vi "Magazine Control 3.0.vi"(0 "Magazine Overflow Power":dbl=1.0, 4 "Magazine Power":dbl=1.0, 6 "Intake Power":dbl=1.0, 8 "Outtake Sensor":bool, 9 "Intake Sensor":bool, 10 "Outtake Button":bool, 11 "Intake Button":bool) -> (2 "Magazine":dbl, 3 "Intake":dbl)   [LabVIEW 2019]
uses:
  Magazine State.ctl
  78d4d847-6c27-4930-b494-8e57f4631178.vi
  83c46ad4-0f57-42ca-80be-7e1131384452.vi
  952471bd-31fd-4431-ad26-f7d2215ef338.vi
panel:
  out "Current State":T1
  in  "Initial State":T1
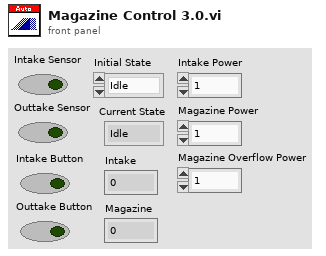
[diagram p1: front panel]
types:
  T1 = typedef "Magazine State.ctl" = enum16{"Idle", "Intake Idle", "Move Cell", "Prevent Overflow", "Outtake Idle", "Shoot"}
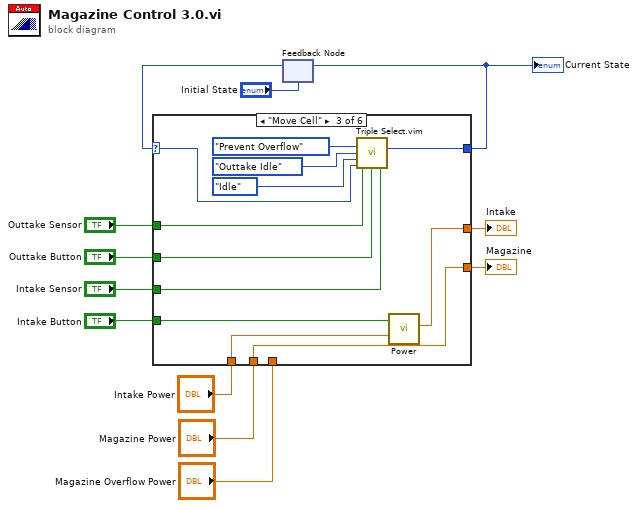
[diagram p0: block diagram]
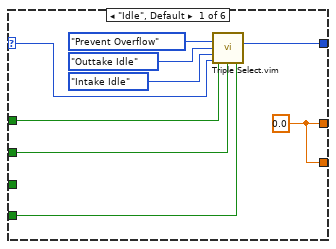
[diagram p2: hidden frame]
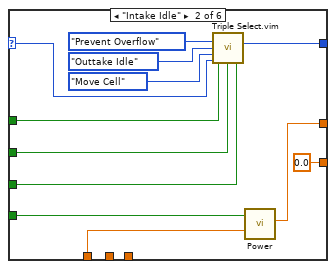
[diagram p3: hidden frame]
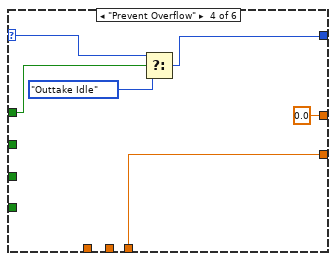
[diagram p4: hidden frame]
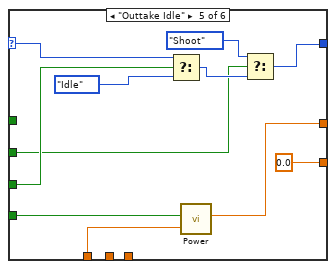
[diagram p5: hidden frame]
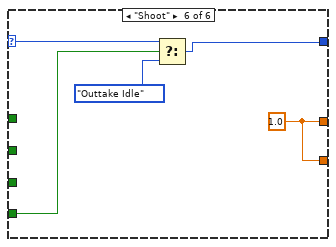
[diagram p6: hidden frame]
diagram:
  n1 = feedback #1("Initial State") -> (w3:T1)
  n2 = case shown="\"Move Cell\"" w3 {
    selector: w3 -> [w13 w27 w39 w49 w58 w66]
    tunnel: "Intake Button" -> [w17 w31 w45 _ w62 w67]
    tunnel: [w21 w33 w44 0.0 ("Output") w61 w63] -> w10
    tunnel: [w21 0.0 w43 w51 0.0 ("Magazine Overflow Power") w63] -> w9
    tunnel: "Intake Power" -> [_ w22 w34 _ w52 _]
    tunnel: "Intake Sensor" -> [_ w24 w36 _ w59 _]
    tunnel: "Magazine Power" -> [_ _ w43 _ _ _]
    tunnel: [w14 w23 w35 w48 w53 w64] -> w1
    tunnel: "Magazine Overflow Power" -> [_ _ _ w51 _ _]
    tunnel: "Outtake Button" -> [w16 w26 w37 _ w55 _]
    tunnel: "Outtake Sensor" -> [w15 w25 w38 w46 _ _]
    frame "Idle", Default {
      w21 = 0.0
      n3 = call "Triple Select.vim"("Input 1"=Magazine_State."Prevent Overflow" ("lower limit"), "Input 2"=Magazine_State."Outtake Idle" ("lower limit"), "Input 3"=Magazine_State."Intake Idle", "Input 4"=w13, "Selection 1"=w15, "Selection 2"=w16, "Selection 3"=w17) -> ("Output"=w14:T1)  [unwired: 8 in]
    }
    frame "Intake Idle" {
      n4 = call "Triple Select.vim"("Input 1"=Magazine_State."Prevent Overflow" ("lower limit"), "Input 2"=Magazine_State."Outtake Idle" ("lower limit"), "Input 3"=Magazine_State."Move Cell", "Input 4"=w27, "Selection 1"=w25, "Selection 2"=w26, "Selection 3"=w24) -> ("Output"=w23:T1)  [unwired: 8 in]
      n5 = call "Power.vi"("Positive Power"=w22, "Positive"=w31) -> ("Output"=w33:dbl)  [unwired: 9 in]
    }
    frame "Move Cell" {
      n6 = call "Triple Select.vim"("Input 1"=Magazine_State."Prevent Overflow" ("lower limit"), "Input 2"=Magazine_State."Outtake Idle" ("lower limit"), "Input 3"=Magazine_State."Idle", "Input 4"=w39, "Selection 1"=w38, "Selection 2"=w37, "Selection 3"=w36) -> ("Output"=w35:T1)  [unwired: 8 in]
      n7 = call "Power.vi"("Positive Power"=w34, "Positive"=w45) -> ("Output"=w44:dbl)  [unwired: 9 in]
    }
    frame "Prevent Overflow" {
      n8 = Select(t=w49, s=w46, f=Magazine_State."Outtake Idle" ("lower limit")) -> (s? t:f=w48:T1)
    }
    frame "Outtake Idle" {
      n9 = Select(t=w58, s=w59, f=Magazine_State."Idle") -> (s? t:f=w56:T1)
      n10 = call "Power.vi"("Positive Power"=w52, "Positive"=w62) -> ("Output"=w61:dbl)  [unwired: 9 in]
      n11 = Select(t=Magazine_State."Shoot" ("f"), s=w55, f=w56) -> (s? t:f=w53:T1)
    }
    frame "Shoot" {
      w63 = 1.0 ("Magazine Overflow Power")
      n12 = Select(t=w66, s=w67, f=Magazine_State."Outtake Idle") -> (s? t:f=w64:T1)
    }
  }
  "Current State" <- w1
  "Intake" <- w10
  "Magazine" <- w9
  n13 = feedback-in #1(w1) -> ()
